vi "File.Check File Path.vi"(8 "error in (no error)":errorcluster, 9 "FileMustExist?":bool, 10 "FileNameSuffixes":string[](array[string]), 11 "PathIn":path) -> (0 "error out":errorcluster, 3 "Path Out":path)   [LabVIEW 2024]
uses:
  Errors/Error.Error Code List.ctl
  <vilib>/KATE/Files/File Utils.lvlib
  Errors.lvlib
  File Utils.lvlib
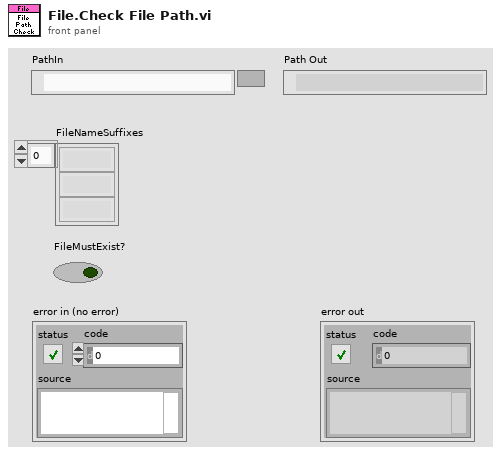
[diagram p1: front panel]
types:
  T1 = typedef "EQMF.lvlib/Errors.lvlib/Error.Error Code List.ctl" = i32
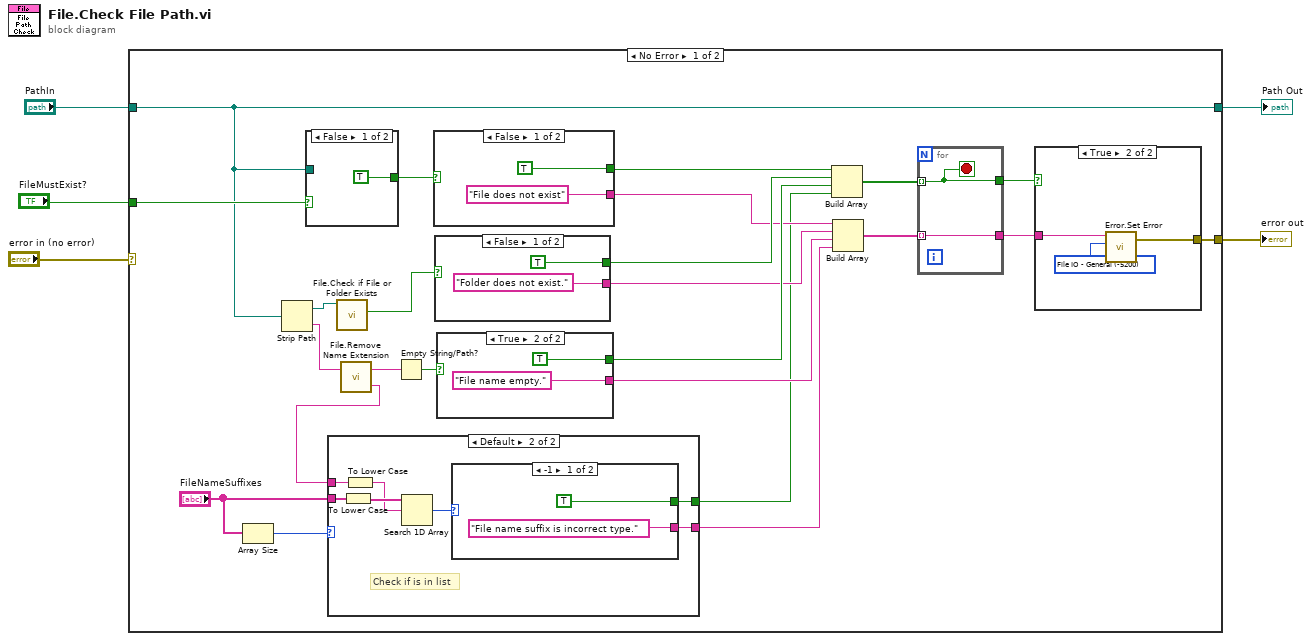
[diagram p0: block diagram]
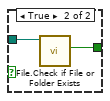
[diagram p5: hidden frame]
diagram:
  n1 = case shown="No Error" "error in (no error)" {
    selector: "error in (no error)" -> [_ w53]
    tunnel: "PathIn" -> [w8 w54]
    tunnel: "FileMustExist?" -> [w23 _]
    tunnel: [w8 w54] -> w3
    tunnel: [w7 w53] -> w1
    frame No Error {
      n2 = Array Size(array="FileNameSuffixes") -> (size(s)=w6:i32)
      n3 = Strip Path(path=w8) -> (stripped path=w29:path, name=w28:string)
      n4 = case shown="False" w23 {
        tunnel: w8 -> [_ w46]
        tunnel: [TRUE w45] -> w24
        frame False {
        }
        frame True {
          n5 = call <vilib>:"File.Check if File or Folder Exists.vi"("Path"=w46) -> ("Exists"=w45:bool)  [unwired: 6 in, 4 out]
        }
      }
      n6 = call <vilib>:"File.Check if File or Folder Exists.vi"("Path"=w29) -> ("Exists"=w25:bool)  [unwired: 6 in, 4 out]
      n7 = call "File.Remove Name Extension.vi"("File Name"=w28) -> ("Ext"=w16:string, "Name Less Ext"=w27:string)  [unwired: 1 in]
      n8 = case shown="Default" w6 {
        tunnel: w16 -> [_ w41]
        tunnel: "FileNameSuffixes" -> [_ w40]
        tunnel: [_ w36] -> w14
        tunnel: [_ w35] -> w13
        frame 0 {
        }
        frame Default {
          # "Check if is in list"
          n9 = To Lower Case(string=w40) -> (all lower case string=w39:string[])
          n10 = To Lower Case(string=w41) -> (all lower case string=w38:string)
          n11 = Search 1D Array(1D array=w39, element=w38) -> (index of element=w37:i32)  [unwired: 1 in]
          n12 = case shown="-1" w37 {
            tunnel: ["File name suffix is incorrect type." _] -> w35
            tunnel: [TRUE _] -> w36
            frame -1 {
            }
            frame Default {
            }
          }
        }
      }
      n13 = Empty String/Path?(string/path=w27) -> (empty?=w26:bool)
      n14 = case shown="False" w24 {
        tunnel: ["File does not exist" _] -> w19
        tunnel: [TRUE _] -> w22
        frame False {
        }
        frame True {
        }
      }
      n15 = case shown="False" w25 {
        tunnel: ["Folder does not exist." _] -> w18
        tunnel: [TRUE _] -> w21
        frame False {
        }
        frame True {
        }
      }
      n16 = case shown="True" w26 {
        tunnel: [_ "File name empty."] -> w17
        tunnel: [_ TRUE] -> w20
        frame False {
        }
        frame True {
        }
      }
      n17 = Build Array(w22, w21, w20, w14) -> (w12:bool[])
      n18 = Build Array(w19, w18, w17, w13) -> (w11:string[])
      n19 = for {
        tunnel: w12 -> [w33] mode=indexing
        tunnel: w11 -> [w34] mode=indexing
        tunnel: [w34] -> w9
        tunnel: [w33] -> w10
        stop <- w33 stop-if-true
      }
      n20 = case shown="True" w10 {
        tunnel: w9 -> [_ w32]
        tunnel: [_ w30] -> w7
        frame False {
        }
        frame True {
          w31 = T1 -5200 items=["No Error"=0, "Abort"=-2, "Misc"=-5000, "Fixture Error"=-5100, "File IO - General"=-5200, "FIle IO - Config Error"=-5201, "Instrument - General"=-5300, "Instrument - Serial Com"=-5301, "Instrument - Camera"=-5302, "Instrument - PS"=-5303, "Instrument - Oscilloscope"=-5304, "Instrument - Function Gen"=-5305, "Instrument - Load"=-5306, "Instrument - Meter"=-5307, "Instrument - Power Control"=-5308, "Instrument - Motion"=-5309, "Instrument - RF"=-5310, "System Exe"=-5400, "Image Processing"=-5500, "Communication"=-5600, "Script - Syntax Error"=-6000, "Script - Invalid Name or Param"=-6100, "Script - Timeout"=-6200, "Invalid Data"=-6300, "FW Update Error"=-6500] ("Std Code")
          n21 = call "Error.Set Error.vi"("Std Code"=w31, "Desc"=w32) -> ("error out"=w30:errorcluster)  [unwired: 5 in]
        }
      }
    }
    frame Error {
    }
  }
  "error out" <- w1
  "Path Out" <- w3
